vi "Get Last Test Status.vi"(8 "error in (no error)":errorcluster, 11 "Results Manager in":refnum<class "Results Manager.lvclass">) -> (0 "error out":errorcluster, 2 "Test Status":T1, 3 "Results Manager out":refnum<class "Results Manager.lvclass">)   [LabVIEW 2021, in "Sequence Engine.lvlib" / "Results Manager.lvclass"]
uses:
  Results Manager.lvclass
  Test Result/Test Status.ctl
  Results Manager.lvclass/Results Manager.ctl
  Test Result/Test Result.lvclass/Test Result.ctl
  Test Result/Test Result.lvclass
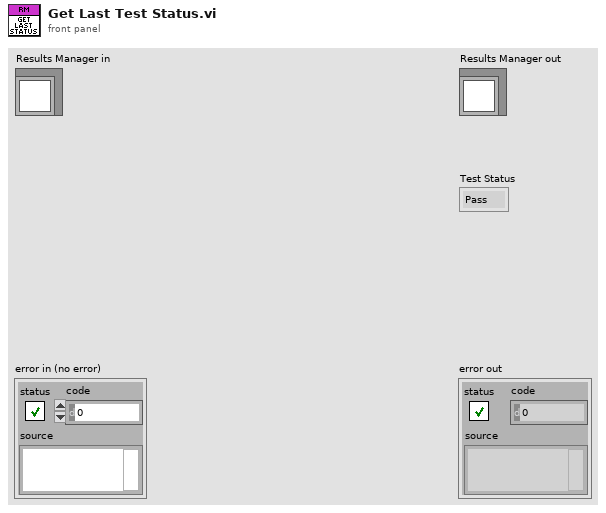
[diagram p1: front panel]
types:
  T1 = typedef "Sequence Engine.lvlib/Test Result.lvclass/Test Status.ctl" = enum16{"Pass", "Fail", "Aborted", "Skipped"}
  T2 = typedef "Sequence Engine.lvlib/Test Result.lvclass/Result Data.ctl" = cluster{"Test ID":u32, "Test Name":string, "Sub Test Name":string, "Test Status":T1, "Start Time":timestamp, "End Time":timestamp, "Duration (s)":dbl, "Expected Values":string, "Measured Values":string, "Remarks":string}
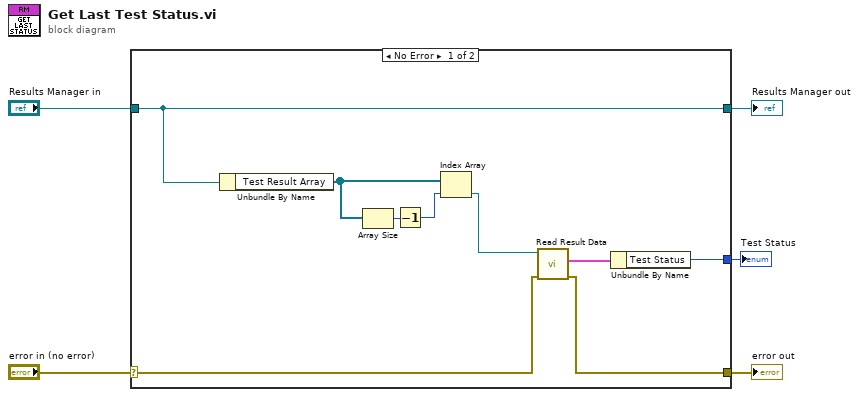
[diagram p0: block diagram]
diagram:
  n1 = case shown="No Error" "error in (no error)" {
    selector: "error in (no error)" -> [w9 w16]
    tunnel: [w8 w16] -> w4
    tunnel: [w14 w15] -> w2
    tunnel: "Results Manager in" -> [w14 w15]
    tunnel: [w6 _] -> w1
    frame No Error {
      n2 = Unbundle By Name(w14) -> ("Test Result Array"=w13:refnum<class "Test Result.lvclass">[])
      n3 = Array Size(array=w13) -> (size(s)=w12:i32)
      n4 = Decrement(x=w12) -> (x-1=w11:i32)
      n5 = Index Array(array=w13, index=w11) -> (element=w10:refnum<class "Test Result.lvclass">)
      n6 = call "Read Result Data.vi"("error in (no error)"=w9, "Test Result in"=w10) -> ("error out"=w8:errorcluster, "Result Data"=w7:T2)  [unwired: 7 in, 1 out]
      n7 = Unbundle By Name(w7) -> ("Test Status"=w6:T1)
    }
    frame Error {
    }
  }
  "error out" <- w4
  "Results Manager out" <- w2
  "Test Status" <- w1
